vi "Subtask 2.vi"() -> ()   [LabVIEW 2016, in "Test.lvrbt"]
uses:
  Test.lvrbt
  <vilib>/NXT/Block Support/NXT_OutputPort.ctl
  <vilib>/NXT/Block Support/NXT_InputPort.ctl
  <vilib>/NXT/Dual Mode Library/Motors/ResetMotor.vi
  <vilib>/NXT/Dual Mode Library/Waits/Wait_Num(msec).vi
  <vilib>/NXT/Dual Mode Library/Display/drawText.vi
  <vilib>/NXT/Dual Mode Library/Sensors/EV3_Color_Reflect.vi
  <vilib>/NXT/Dual Mode Library/Sensors/Touch_Pressed.vi
  <vilib>/NXT/Dual Mode Library/Sensors/EV3_Ultrasonic_CM.vi
  <vilib>/NXT/Dual Mode Library/Motors/Rotation.vi
  <vilib>/NXT/NXTIO Xnodes/NXTIONodeSubVIs/NXTMoveMotors.vi
  <vilib>/NXT/NXTIO Xnodes/NXTIONodeSubVIs/NXTMotorRunDistance.vi
  <vilib>/NXT/Dual Mode Library/Display/drawNumber.vi
  <vilib>/NXT/NXTIO Xnodes/NXTIONodeSubVIs/NXTMotorSteeringOn.vi
  <vilib>/NXT/NXTIO Xnodes/AddressXNode/NXTIOAddress.xnode
  <vilib>/NXT/Subs/LVHSConnector.ctl
  <vilib>/NXT/NXTIO Xnodes/NXTIOXNode/NXTIO.xnode
  <vilib>/NXT/LegoClasses/BrickReference/BrickReference.lvclass
panel:
  out "kD":dbl(graph)
  out "kI":dbl(graph)
  out "kP":sgl(graph)
  out "Combined":dbl(graph)
  out "Power Sum":dbl
  out "power":dbl
  out "rotation":dbl
  out "button":bool
  out "Distance":dbl
  out "Box Number":dbl
  out "Zone Detector":dbl
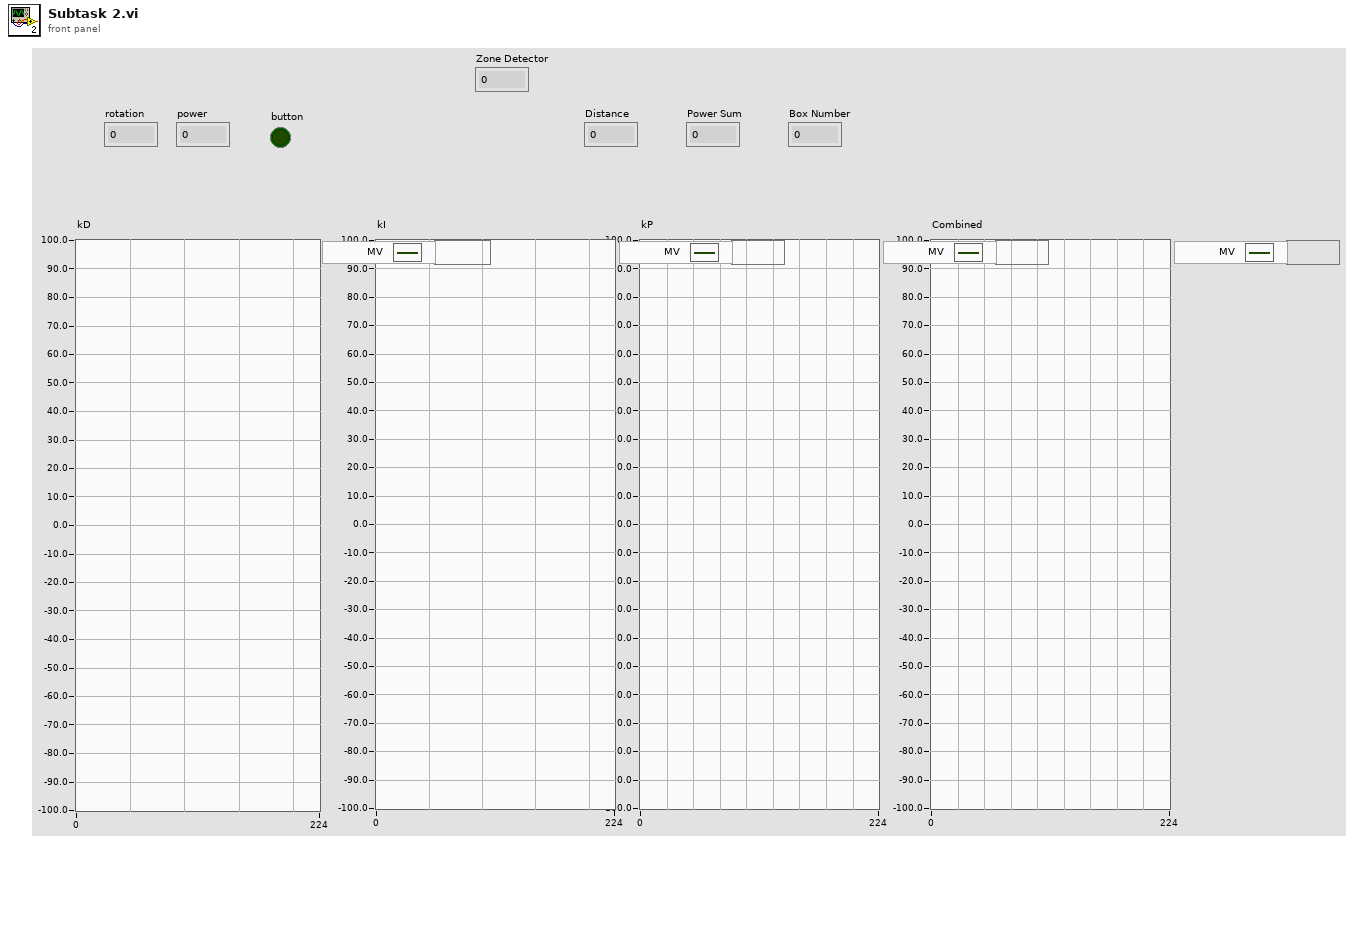
[diagram p1: front panel]
types:
  T1 = typedef "NXT_OutputPort.ctl" = u8
  T2 = typedef "NXT_InputPort.ctl" = u32
  T3 = typedef "LVHSConnector.ctl" = refnum<class "BrickReference.lvclass">
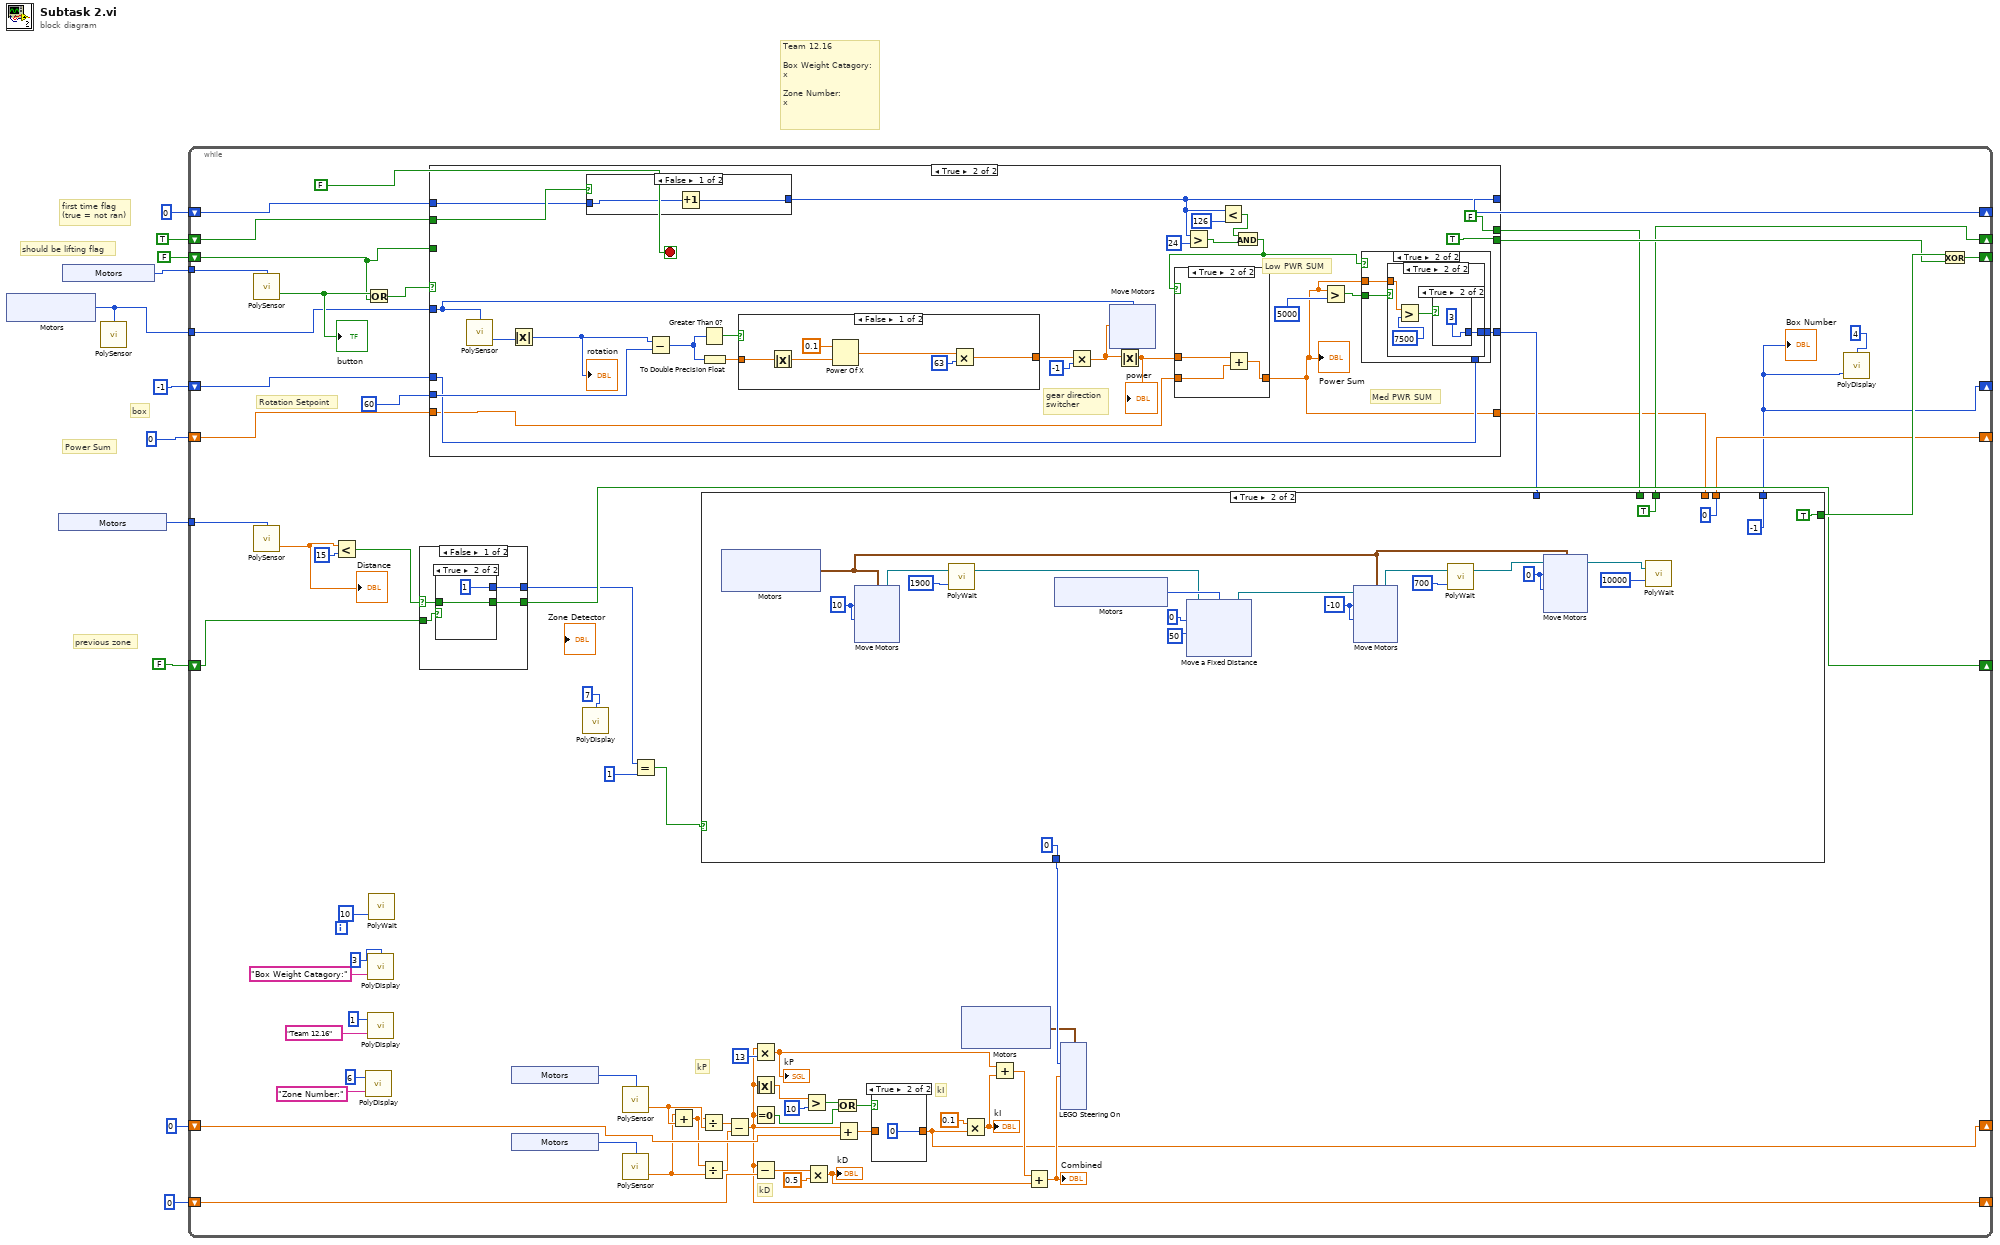
[diagram p0: block diagram]
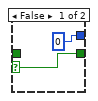
[diagram p2: hidden frame]
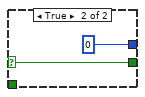
[diagram p3: hidden frame]
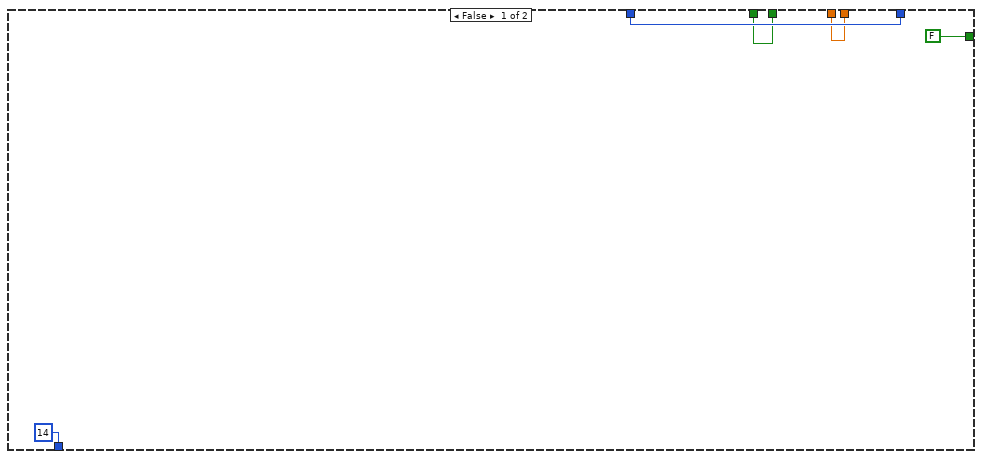
[diagram p4: hidden frame]
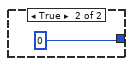
[diagram p6: hidden frame]
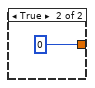
[diagram p8: hidden frame]
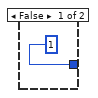
[diagram p10: hidden frame]
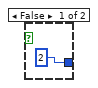
[diagram p11: hidden frame]
diagram:
  # "box"
  # "previous zone"
  # "Team 12.16\n\nBox Weight Catagory:\nx\n\nZone Number:\nx"
  # "should be lifting flag"
  # "first time flag\n(true = not ran)"
  # "Power Sum"
  n1 = xnode "Motors"() -> ("Motor"=w1:T1)
  n2 = xnode "Motors"() -> ("Sensor"=w8:T2)
  n3 = xnode "Motors"() -> ("Sensor"=w7:T2)
  n4 = call-poly <vilib>:"PolySensor.vi"("Port (All Ports)"=w1) -> ()  [unwired: 3 in, 1 out]
  n5 = while {
    shift-right: [w50] -> _
    shift-left: 0 -> [w77]
    shift-right: [w51] -> _
    shift-left: 0 -> [w76]
    tunnel: w1 -> [w32]
    shift-right: [w48] -> _
    shift-left: FALSE -> [w44]
    tunnel: w8 -> [w41]
    tunnel: w7 -> [w42]
    shift-right: [w14] -> _
    shift-left: -1 -> [w40]
    shift-right: [w18] -> _
    shift-left: TRUE -> [w39]
    shift-right: [w16] -> _
    shift-left: 0 -> [w36]
    shift-right: [w34] -> _
    shift-left: u32 0 ("Time (100 msec)") -> [w35]
    shift-right: [w21] -> _
    shift-left: FALSE -> [w22]
    stop <- FALSE stop-if-true
    # "Rotation Setpoint"
    # "kD"
    # "kI"
    # "kP"
    n6 = call-poly <vilib>:"PolySensor.vi"("Port (Port 1)"=w42) -> ("Yes / No"=w53:bool)  [unwired: 2 in, 1 out]
    "button" <- w53
    n7 = call-poly <vilib>:"PolySensor.vi"("Port (Port 1)"=w41) -> ("Centimeters"=w38:sgl)  [unwired: 2 in, 1 out]
    "Distance" <- w38
    n8 = Less?(x=w38, y=15) -> (x < y?=w23:bool)
    n9 = call-poly <vilib>:"PolyDisplay.vi"("Text"="Zone Number:", "Line"=6 ("number")) -> ()  [unwired: 2 in, 1 out]
    n10 = Or(x=w53, y=w44) -> (x .or. y?=w52:bool)
    n11 = call-poly <vilib>:"PolyDisplay.vi"("Text"="Box Weight Catagory:", "Line"=3 ("number")) -> ()  [unwired: 2 in, 1 out]
    n12 = call-poly <vilib>:"PolyDisplay.vi"("Text"="Team 12.16", "Line"=1 ("number")) -> ()  [unwired: 2 in, 1 out]
    n13 = call-poly <vilib>:"PolyWait.vi"("Time (100 msec)"=u32 10) -> ()  [unwired: 3 in, 1 out]
    n14 = case shown="False" w23 {
      selector: w23 -> [w80 w88]
      tunnel: w22 -> [w82 _]
      tunnel: [w81 w88] -> w21
      tunnel: [w79 0] -> w13
      frame False {
        n15 = case shown="True" w82 {
          selector: w82 -> [w84 _]
          tunnel: [w84 w86] -> w81
          tunnel: w80 -> [_ w86]
          tunnel: [0 1] -> w79
          frame False {
          }
          frame True {
          }
        }
      }
      frame True {
      }
    }
    n16 = case shown="True" w52 {
      tunnel: w32 -> [_ w182]
      tunnel: 60 -> [_ w181]
      tunnel: [w155 TRUE] -> w45
      tunnel: w44 -> [w155 _]
      tunnel: [w154 w177] -> w19
      tunnel: w40 -> [w154 w176]
      tunnel: [w153 FALSE] -> w17
      tunnel: w39 -> [w153 w169]
      tunnel: w36 -> [w152 w171]
      tunnel: [w152 w170] -> w15
      tunnel: w35 -> [w151 w168]
      tunnel: [w151 w167] -> w34
      frame False {
      }
      frame True {
        # "gear direction\nswitcher"
        # "Med PWR SUM"
        # "Low PWR SUM"
        n17 = call-poly <vilib>:"PolySensor.vi"("Port (Port A)"=w182) -> ("Angle of Rotation"=w163:i32)  [unwired: 2 in, 1 out]
        n18 = Absolute Value(x=w163) -> (abs(x)=w162:i32)
        "rotation" <- w162
        n19 = case shown="False" w169 {
          tunnel: [w183 u32 0 ("Time (100 msec)")] -> w167
          tunnel: w168 -> [w184 _]
          frame False {
            n20 = Increment(x=w184) -> (x+1=w183:u32)
          }
          frame True {
          }
        }
        n21 = Subtract(x=w162, y=w181) -> (x-y=w175:i32)
        n22 = Greater Than 0?(x=w175) -> (x > 0?=w174:bool)
        n23 = To Double Precision Float(number=w175) -> (double precision float=w173:dbl)
        n24 = case shown="False" w174 {
          tunnel: [w192 0] -> w159
          tunnel: w173 -> [w191 _]
          frame False {
            n25 = Absolute Value(x=w191) -> (abs(x)=w190:dbl)
            n26 = Power Of X(1:w190, 2:0.1) -> (0:w193:dbl)
            n27 = Multiply(x=w193, y=63) -> (x*y=w192:dbl)
          }
          frame True {
          }
        }
        n28 = Multiply(x=w159, y=-1) -> (x*y=w158:dbl)
        n29 = xnode "Move Motors"("Power/Speed 1"=w158, "Motors"=w182) -> ()  [unwired: 1 in, 1 out]
        n30 = Absolute Value(x=w158) -> (abs(x)=w161:dbl)
        "power" <- w161
        n31 = Greater?(x=w167, y=24) -> (0:w164:bool)
        n32 = Less?(x=w167, y=126) -> (x < y?=w165:bool)
        n33 = And(x=w165, y=w164) -> (x .and. y?=w156:bool)
        n34 = case shown="True" w156 {
          tunnel: w161 -> [_ w189]
          tunnel: [w186 w188] -> w170
          tunnel: w171 -> [w186 w187]
          frame False {
          }
          frame True {
            n35 = Add(x=w189, y=w187) -> (x+y=w188:dbl)
          }
        }
        "Power Sum" <- w170
        n36 = Greater?(x=w170, y=5000) -> (0:w179:bool)
        n37 = case shown="True" w156 {
          tunnel: w179 -> [_ w207]
          tunnel: [w204 w206] -> w177
          tunnel: w170 -> [_ w205]
          tunnel: w176 -> [w204 _]
          frame False {
          }
          frame True {
            n38 = case shown="True" w207 {
              tunnel: [1 w209] -> w206
              tunnel: w205 -> [_ w211]
              frame False {
              }
              frame True {
                n39 = Greater?(x=w211, y=7500) -> (0:w212:bool)
                n40 = case shown="True" w212 {
                  tunnel: [2 3] -> w209
                  frame False {
                  }
                  frame True {
                  }
                }
              }
            }
          }
        }
      }
    }
    n41 = xnode "Motors"() -> ("Sensor"=w46:T2)
    n42 = xnode "Motors"() -> ("Sensor"=w75:T2)
    n43 = call-poly <vilib>:"PolyDisplay.vi"("Line"=7 ("number")) -> ()  [unwired: 3 in, 1 out]
    n44 = call-poly <vilib>:"PolySensor.vi"("Port (Port 1)"=w46) -> ("Scaled Value"=w74:sgl)  [unwired: 2 in, 1 out]
    n45 = call-poly <vilib>:"PolySensor.vi"("Port (Port 1)"=w75) -> ("Scaled Value"=w73:sgl)  [unwired: 2 in, 1 out]
    n46 = Equal?(x=w13, y=1) -> (x = y?=w37:bool)
    n47 = Add(x=w73, y=w74) -> (x+y=w72:sgl)
    n48 = Divide(x=w72, y=w74) -> (x/y=w71:sgl)
    n49 = Divide(x=w72, y=w73) -> (x/y=w69:sgl)
    n50 = case shown="True" w37 {
      tunnel: [FALSE TRUE] -> w47
      tunnel: [14 0] -> w31
      tunnel: [w91 -1] -> w14
      tunnel: w19 -> [w91 _]
      tunnel: [w90 TRUE] -> w18
      tunnel: w17 -> [w90 _]
      tunnel: [w89 0] -> w16
      tunnel: w15 -> [w89 _]
      frame False {
      }
      frame True {
        w97 = i8 0 ("Power/Speed 2")
        w106 = i8 -10 ("Power/Speed 2")
        w107 = i8 10 ("Power/Speed 2")
        n51 = xnode "Motors"() -> ("Motor"=w98:cluster{"Port":T1, "Port":T1})
        n52 = xnode "Move Motors"("Power/Speed 2"=w107, "Power/Speed 1"=w107, "Motors"=w98) -> ("NXT/EV3"=w112:T3)  [unwired: 1 in]
        n53 = call-poly <vilib>:"PolyWait.vi"("Time (100 msec)"=u32 1900, "NXT/EV3"=w112) -> ("NXT/EV3"=w100:T3)  [unwired: 2 in]
        n54 = xnode "Motors"() -> ("Motor"=w110:T1)
        n55 = xnode "Move a Fixed Distance"("Speed 1"=i8 50 ("Power/Speed 2"), "Distance 1"=i8 0 ("Power/Speed 2"), "Motors"=w110, "NXT/EV3"=w100) -> ("NXT/EV3"=w99:T3)
        n56 = xnode "Move Motors"("Power/Speed 2"=w106, "Power/Speed 1"=w106, "Motors"=w98, "NXT/EV3"=w99) -> ("NXT/EV3"=w104:T3)
        n57 = call-poly <vilib>:"PolyWait.vi"("Time (100 msec)"=u32 700, "NXT/EV3"=w104) -> ("NXT/EV3"=w96:T3)  [unwired: 2 in]
        n58 = xnode "Move Motors"("Power/Speed 2"=w97, "Power/Speed 1"=w97, "Motors"=w98, "NXT/EV3"=w96) -> ("NXT/EV3"=w95:T3)
        n59 = call-poly <vilib>:"PolyWait.vi"("Time (100 msec)"=u32 10000, "NXT/EV3"=w95) -> ()  [unwired: 2 in, 1 out]
      }
    }
    "Box Number" <- w14
    n60 = Subtract(x=w71, y=w69) -> (x-y=w51:sgl)
    n61 = Multiply(x=w51, y=13) -> (x*y=w56:sgl)
    "kP" <- w56
    n62 = Absolute Value(x=w51) -> (abs(x)=w64:sgl)
    n63 = Equal To 0?(x=w51) -> (x = 0?=w66:bool)
    n64 = Subtract(x=w51, y=w76) -> (x-y=w61:sgl)
    n65 = Greater?(x=w64, y=10) -> (0:w63:bool)
    n66 = Multiply(x=w61, y=0.5) -> (x*y=w58:dbl)
    "kD" <- w58
    n67 = Or(x=w63, y=w66) -> (x .or. y?=w65:bool)
    n68 = Add(x=w51, y=w77) -> (x+y=w68:sgl)
    n69 = case shown="True" w65 {
      tunnel: w68 -> [w215 _]
      tunnel: [w215 0] -> w50
      frame False {
      }
      frame True {
      }
    }
    n70 = xnode "Motors"() -> ("Motor"=w20:cluster{"Port":T1, "Port":T1})
    n71 = Multiply(x=0.1, y=w50) -> (x*y=w57:dbl)
    "kI" <- w57
    n72 = Add(x=w56, y=w57) -> (x+y=w59:dbl)
    n73 = Add(x=w59, y=w58) -> (x+y=w55:dbl)
    "Combined" <- w55
    n74 = xnode "LEGO Steering On"("Steering 1"=w55, "Power 1"=w31, "Motors"=w20) -> ()  [unwired: 1 in, 1 out]
    n75 = call-poly <vilib>:"PolyDisplay.vi"("number"=w14, "Line"=4 ("number")) -> ()  [unwired: 2 in, 1 out]
    n76 = Exclusive Or(1:w45, 2:w47) -> (0:w48:bool)
  }
